vi "point_to_time_4(SubVI).vi"(9 "number of points":i32, 10 "DAC frequency(MHz)":dbl, 11 "point location":i32) -> (1 "dt (us)":dbl, 2 "Pulse Width (us)":dbl, 3 "time (us)":dbl)   [LabVIEW 2016]
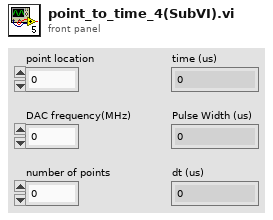
[diagram p1: front panel]
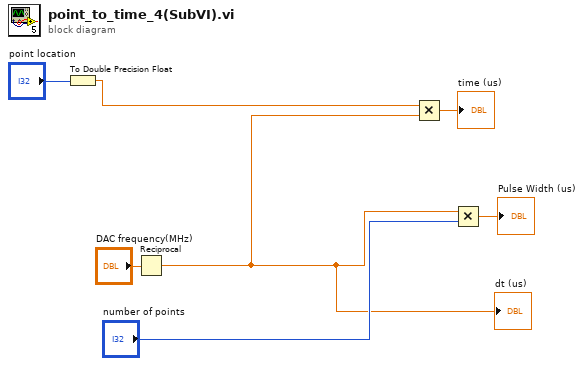
[diagram p0: block diagram]
diagram:
  n1 = To Double Precision Float(number="point location") -> (double precision float=w2:dbl)
  n2 = Reciprocal(x="DAC frequency(MHz)") -> (1/x=w1:dbl)
  "dt (us)" <- w1
  n3 = Multiply(x=w2, y=w1) -> (x*y=→"time (us)":dbl)
  n4 = Multiply(x=w1, y="number of points") -> (x*y=→"Pulse Width (us)":dbl)
